vi "Read Rx Channel.vi"(8 "error in":errorcluster, 9 "labels settings for RT":T1[](array[typedef]) {"Label Timestamp Channel Data Reference" format="%.0x"; "Word Initial Raw Value" format="%032.0f"; "Label Disable/Trigger Channel Reference" format="%.0x"; "parameter driver data"."Tx parameter refs" format="%.0x"; "SDI" format="%02b"; "label" format="%.0o"}, 10 "channel number in":u8, 11 "board handle in":u8) -> (0 "error out":errorcluster, 1 "data out":u32[](array[numeric]), 2 "channel number out":u8, 3 "board handle out":u8)   [LabVIEW 2020, in "AIM ARINC 429 Hardware API.lvlib"]
uses:
  AIM ARINC 429 Hardware API.lvlib
  Shared/RT Label Settings.ctl
  Shared/Label.ctl
  Shared/RT Parameters.ctl
  Shared/Parameter Definition.ctl
  <vilib>/NI/NI VeriStand Encoding and Decoding/Encoding.ctl
  <vilib>/NI VeriStand/Custom Device API/Custom Device Item Ref.ctl
  Shared/Transfer Type.ctl
  <vilib>/NI VeriStand/Custom Device API/Data Reference.ctl
  <instrlib>/AIM GmbH/_ARINC-429/subvi/Error Converter (ErrCode or Status).vi
  <instrlib>/AIM GmbH/_ARINC-429/subvi/Get Library Path.vi
  <instrlib>/AIM GmbH/_ARINC-429/VIs/Library/Api429Lib Error Desc Get.vi
  <instrlib>/AIM GmbH/_ARINC-429/subvi/Get Error Number Offset.vi
  <vilib>/Utility/error.llb/Error Cluster From Error Code.vi
  <instrlib>/AIM GmbH/_ARINC-429/AIM429LV.lvlib
  <vilib>/NI/NI VeriStand Encoding and Decoding/Encoding and Decoding.lvlib
  <vilib>/NI VeriStand/Custom Device API/Custom Device API.lvlib
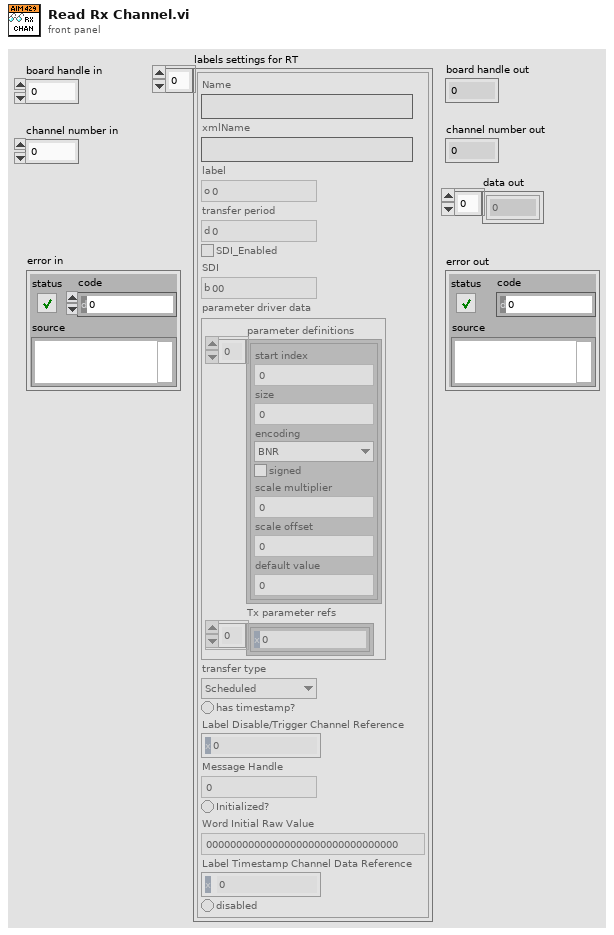
[diagram p1: front panel]
types:
  T1 = typedef "RT Label Settings.ctl" = cluster{"Name":string, "xmlName":string, "label":T2, "transfer period":u32, "SDI_Enabled":bool, "SDI":u8, "parameter driver data":T3, "transfer type":T7, "has timestamp?":bool, "Label Disable/Trigger Channel Reference":T6, "Message Handle":u64, "Initialized?":bool, "Word Initial Raw Value":u32, "Label Timestamp Channel Data Reference":T8, "disabled":bool}
  T2 = typedef "Label.ctl" = u8
  T3 = typedef "RT Parameters.ctl" = cluster{"parameter definitions":T4[], "Tx parameter refs":T6[]}
  T4 = typedef "Parameter Definition.ctl" = cluster{"start index":i32, "size":i32, "encoding":T5, "signed":bool, "scale multiplier":dbl, "scale offset":dbl, "default value":dbl}
  T5 = typedef "Encoding and Decoding.lvlib/Encoding.ctl" = enum16{"BNR", "BCD", "Discrete"}
  T6 = typedef "Custom Device API.lvlib/Custom Device Item Ref.ctl" = u64
  T7 = typedef "Transfer Type.ctl" = enum16{"Scheduled", "Acyclic", "Block", "Strobe"}
  T8 = typedef "Custom Device API.lvlib/Data Reference.ctl" = i32
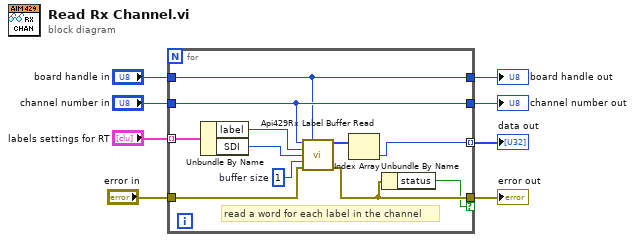
[diagram p0: block diagram]
diagram:
  n1 = for {
    tunnel: "channel number in" -> [w13]
    tunnel: "board handle in" -> [w12]
    tunnel: "labels settings for RT" -> [w19] mode=indexing
    tunnel: [w11] -> w3 mode=indexing
    tunnel: [w13] -> w2
    tunnel: [w12] -> w1
    tunnel: "error in" -> [w15]
    tunnel: [w10] -> w4 if=w9
    w16 = u16 1  # buffer size
    # "read a word for each label in the channel"
    n2 = Unbundle By Name(w19) -> ("label"=w17:T2, "SDI"=w18:u8)
    n3 = call <instrlib>:"Api429Rx Label Buffer Read.vi"("b_Chn"=w13, "board_handle"=w12, "b_Label"=w17, "b_Sdi"=w18, "w_BufSize"=w16, "error in (no error)"=w15) -> ("px_LData out"=w14:u32[], "error out"=w10:errorcluster)  [unwired: 7 in, 1 out]
    n4 = Index Array(array=w14) -> (element=w11:u32)  [unwired: 1 in]
    n5 = Unbundle By Name(w10) -> ("status"=w9:bool)
  }
  "board handle out" <- w1
  "channel number out" <- w2
  "error out" <- w4
  "data out" <- w3
